vi "Stop Acquisition.vi"(8 "error in (no error)":errorcluster, 11 "Hardware Resources in":T1) -> (0 "error out":errorcluster)   [LabVIEW 2018, in "DAQ.lvlib"]
doc: "Stops the acquisition."
uses:
  Hardware Configuration.ctl
  Task Cluster.ctl
  DAQ/DAQ.lvlib
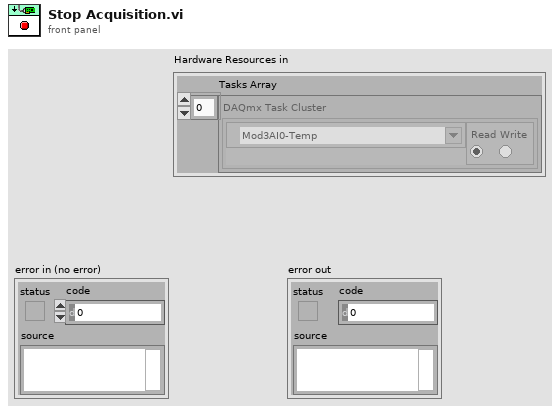
[diagram p1: front panel]
types:
  T1 = typedef "DAQ.lvlib/Hardware Configuration.ctl" = cluster{"Tasks Array":T2[]}
  T2 = typedef "Task Cluster.ctl" = cluster{"DAQmx Task":refnum<k21>, "Read-Write Radio":enum32{"Read", "Write"}}
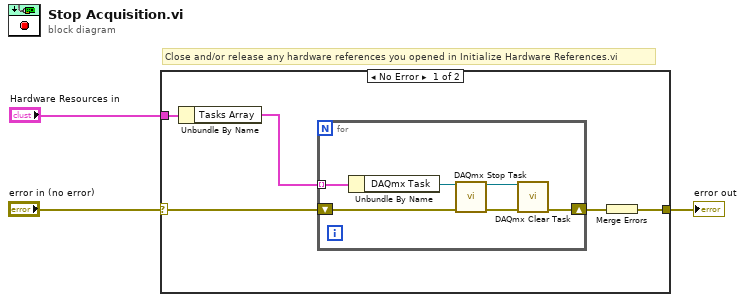
[diagram p0: block diagram]
diagram:
  # "Close and/or release any hardware references you opened in Initialize Hardware References.vi"
  n1 = case shown="No Error" "error in (no error)" {
    selector: "error in (no error)" -> [w6 w15]
    tunnel: [w8 w15] -> w2
    tunnel: "Hardware Resources in" -> [w7 _]
    frame No Error {
      n2 = Unbundle By Name(w7) -> ("Tasks Array"=w5:T2[])
      n3 = for {
        tunnel: w5 -> [w13] mode=indexing
        shift-right: [w10] -> w4
        shift-left: w6 -> [w14]
        n4 = Unbundle By Name(w13) -> ("DAQmx Task"=w9:refnum<k21>)
        n5 = call <vilib>:"DAQmx Stop Task.vi"("task/channels in"=w9, "error in"=w14) -> ("task out"=w12:refnum<k21>, "error out"=w11:errorcluster)  [unwired: 12 in]
        n6 = call <vilib>:"DAQmx Clear Task.vi"("task in"=w12, "error in"=w11) -> ("error out"=w10:errorcluster)  [unwired: 13 in]
      }
      n7 = Merge Errors(w4) -> (w8:errorcluster)
    }
    frame Error {
    }
  }
  "error out" <- w2
